vi "Query Flow Coefficient.vi"(8 "error in (no error)":errorcluster, 11 "VISA resource name":refnum<visa-resource-name>) -> (0 "error out":errorcluster, 2 "Flow Coefficient":dbl, 3 "VISA resource name out":refnum<visa-resource-name>)   [LabVIEW 2023, in "Fluke Molbox 1 Plus.lvlib"]
doc: "Queries the molbox1+ for the flow coefficient. The flow coefficent is a value that is ued to convert kg/s to the current flow units. It is dependent on the current flow unit and the gas selected. To use this coefficient, multiply it by kg/s to get flow in the current flow units."
uses:
  Fluke Molbox 1 Plus.lvlib
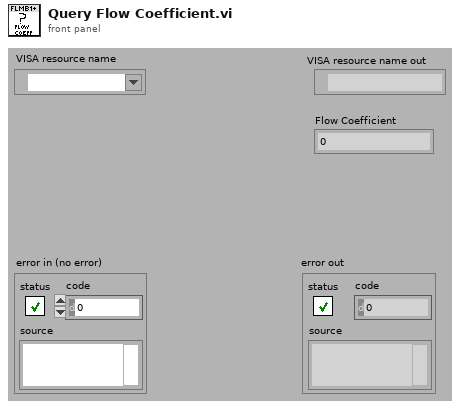
[diagram p1: front panel]
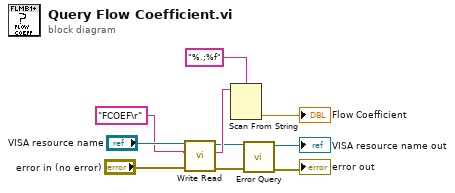
[diagram p0: block diagram]
diagram:
  n1 = call "Write Read.vi"("error in (no error)"="error in (no error)", "Write String"="FCOEF\r" ("write buffer"), "VISA resource name"="VISA resource name") -> ("error out"=w3:errorcluster, "Read Response"=w5:string, "VISA resource name out"=w4:refnum<visa-resource-name>)  [unwired: 6 in]
  n2 = Scan From String(format string="%.;%f", input string=w5) -> (output 1=→"Flow Coefficient":dbl)  [unwired: 3 in, 3 out]
  n3 = call "Error Query.vi"("error in (no error)"=w3, "VISA resource name"=w4) -> ("error out"=→"error out":errorcluster, "VISA resource name out"=→"VISA resource name out":refnum<visa-resource-name>)  [unwired: 6 in, 2 out]
